vi "Initialize Object.vi"(8 "error in (no error)":errorcluster, 9 "Object Cluster In":T1) -> (0 "error out":errorcluster, 1 "Object Cluster Out":T1)   [LabVIEW 2020, in "3D Plot.lvclass"]
uses:
  <vilib>/Math Plots/3D Math Plots/3D Plot/3D Plot/3D Plot.lvclass
  <vilib>/Math Plots/3D Math Plots/3D Plot/3D Plot/Typedef/Object Cluster.ctl
  <vilib>/picture/3D Picture Control/Object/Create Object (name).vi
  <vilib>/picture/3D Picture Control/NI_3D Picture Control.lvlib
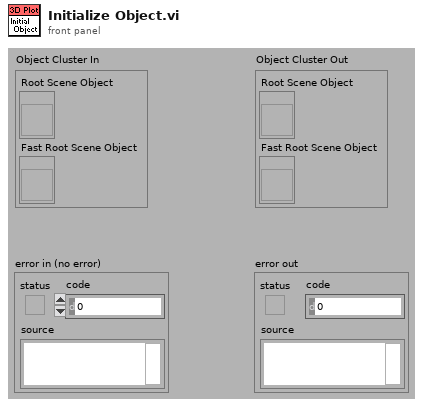
[diagram p1: front panel]
types:
  T1 = typedef "3D Plot.lvclass/Object Cluster.ctl" = cluster{"Root Scene Object":refnum<vi>, "Fast Root Scene Object":refnum<vi>}
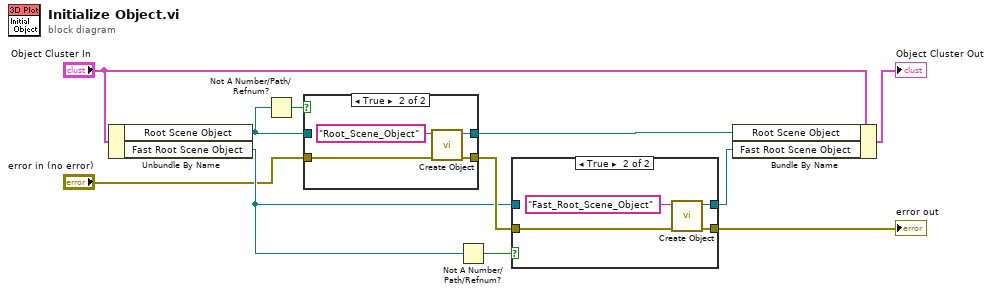
[diagram p0: block diagram]
diagram:
  n1 = Unbundle By Name("Object Cluster In") -> ("Root Scene Object"=w6:refnum<vi>, "Fast Root Scene Object"=w5:refnum<vi>)
  n2 = Not A Number/Path/Refnum?(number/path/refnum=w6) -> (NaN/Path/Refnum?=w9:bool)
  n3 = case shown="True" w9 {
    tunnel: w6 -> [w13 _]
    tunnel: [w13 w15] -> w3
    tunnel: [w12 w14] -> w10
    tunnel: "error in (no error)" -> [w12 w17]
    frame False {
    }
    frame True {
      n4 = call-poly <vilib>:"Create Object.vi"("error in (no error)"=w17, "Name"="Root_Scene_Object") -> ("error out"=w14:errorcluster, "Scene:New Object"=w15:refnum<vi>)  [unwired: 8 in]
    }
  }
  n5 = Not A Number/Path/Refnum?(number/path/refnum=w5) -> (NaN/Path/Refnum?=w11:bool)
  n6 = case shown="True" w11 {
    tunnel: w5 -> [w19 _]
    tunnel: [w19 w21] -> w2
    tunnel: [w18 w20] -> w1
    tunnel: w10 -> [w18 w23]
    frame False {
    }
    frame True {
      n7 = call-poly <vilib>:"Create Object.vi"("error in (no error)"=w23, "Name"="Fast_Root_Scene_Object") -> ("error out"=w20:errorcluster, "Scene:New Object"=w21:refnum<vi>)  [unwired: 8 in]
    }
  }
  "error out" <- w1
  n8 = Bundle By Name(cluster="Object Cluster In", "Root Scene Object"=w3, "Fast Root Scene Object"=w2) -> (→"Object Cluster Out":T1)
